vi "Clear Console.vi"(7 "Clear Logfile":bool, 8 "error in (no error)":errorcluster, 11 "Console Log in":refnum<class "Console Log.lvclass">) -> (0 "error out":errorcluster, 3 "Console Log out":refnum<class "Console Log.lvclass">)   [LabVIEW 2023, in "Console Log.lvclass"]
uses:
  Console Log.lvclass
  Console Log.lvclass/Console Log.ctl
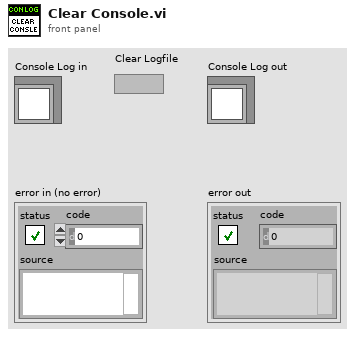
[diagram p1: front panel]
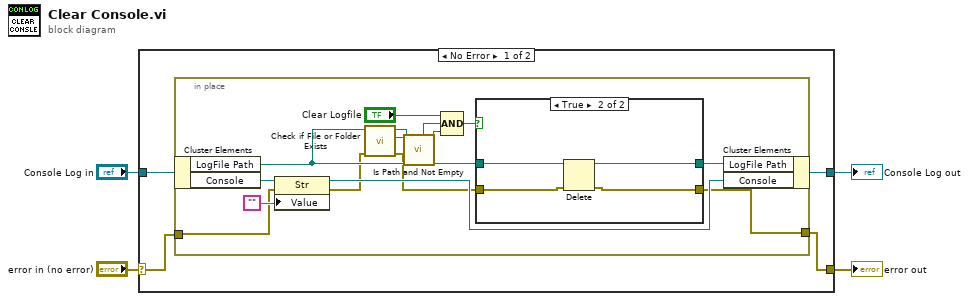
[diagram p0: block diagram]
diagram:
  n1 = case shown="No Error" "error in (no error)" {
    selector: "error in (no error)" -> [w8 w30]
    tunnel: [w5 w30] -> w3
    tunnel: [w6 w29] -> w1
    tunnel: "Console Log in" -> [w7 w29]
    frame No Error {
      n2 = in-place {
        in-place-border: w8 -> [w20]
        in-place-border: [w17] -> w5
        n3 = in-place-cluster #1(w7) -> ("LogFile Path"=w16:path, "Console"=w22:refnum<vi>)
        n4 = property class="Str"(reference=w22, error in=w20, "Value"="") -> (reference out=w19:refnum<vi>, error out=w15:errorcluster)
        n5 = call <vilib>:"Check if File or Folder Exists.vi"("error in (no error)"=w15, "path"=w16) -> ("error out"=w14:errorcluster, "file or folder exists?"=w12:bool, "dup path"=w10:path)  [unwired: 7 in]
        n6 = call <vilib>:"Is Path and Not Empty.vi"("path"=w10) -> ("Is Path and Not Empty?"=w9:bool)  [unwired: 4 in]
        n7 = Compound Arithmetic op=AND("Clear Logfile", w12, w9) -> (w11:bool)
        n8 = case shown="True" w11 {
          tunnel: w14 -> [w23 w27]
          tunnel: w16 -> [w24 w28]
          tunnel: [w24 w25] -> w18
          tunnel: [w23 w26] -> w17
          frame False {
          }
          frame True {
            n9 = Delete(path (use dialog)=w28, error in=w27) -> (deleted path=w25:path, error out=w26:errorcluster)  [unwired: 3 in, 1 out]
          }
        }
        n10 = in-place-cluster #1("LogFile Path"=w18, "Console"=w19) -> (w6:refnum<class "Console Log.lvclass">)
      }
    }
    frame Error {
    }
  }
  "error out" <- w3
  "Console Log out" <- w1
